vi "SMTP Email MIME Send File Attachment.vi"(4 "MIME content-type":string, 5 "translit":string, 6 "binary (F)":bool, 7 "character set":string, 8 "error in (no error)":errorcluster, 9 "name (file name)":string, 10 "path":path, 11 "smtp session":T1) -> (0 "error out":errorcluster, 2 "file error":errorcluster, 3 "smtp session out":T1)   [LabVIEW 2009, in "NewNI_SMTPEmail.lvlib"]
uses:
  NewNI_SMTPEmail.lvlib
  SMTP Email Session.ctl
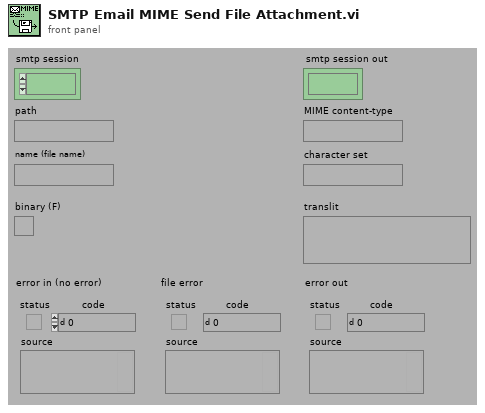
[diagram p1: front panel]
types:
  T1 = typedef "NewNI_SMTPEmail.lvlib/SMTP Email Session.ctl" = refnum<k1>
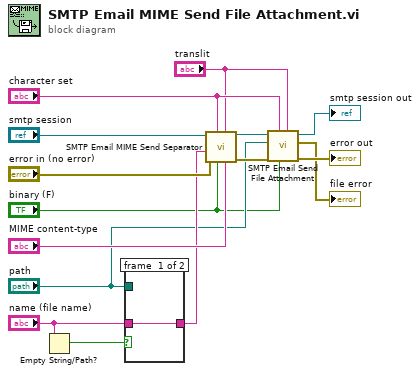
[diagram p0: block diagram]
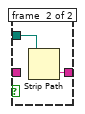
[diagram p2: hidden frame]
diagram:
  n1 = Empty String/Path?(string/path="name (file name)") -> (empty?=w12:bool)
  n2 = case shown="True" w12 {
    tunnel: "name (file name)" -> [w16 _]
    tunnel: [w16 w18] -> w11
    tunnel: "path" -> [_ w17]
    frame #0 {
    }
    frame #1 {
      n3 = Strip Path(path=w17) -> (name=w18:string)  [unwired: 1 out]
    }
  }
  n4 = call "SMTP Email MIME Send Separator.vi"("MIME content-type"="MIME content-type", "translit"="translit", "binary (F)"="binary (F)", "character set"="character set", "error in (no error)"="error in (no error)", "name"=w11, "smtp session"="smtp session") -> ("error out"=w9:errorcluster, "smtp session out"=w7:T1)  [unwired: 1 in, 2 out]
  n5 = call "SMTP Email Send File Attachment.vi"("translit"="translit", "binary? (F)"="binary (F)", "character set"="character set", "error in (no error)"=w9, "path"="path", "smtp session"=w7) -> ("error out"=→"error out":errorcluster, "file error"=→"file error":errorcluster, "smtp session out"=→"smtp session out":T1)  [unwired: 3 out]
